vi "Power Supply (No Objects).vi"(8 "error in (no error)":errorcluster, 11 "Cluster In":T4={"Field"=0.0, "Rate"=0.0, "Status"={"Sweeping"=FALSE, "Clamped"=FALSE, "Hold"=FALSE, "At Rest"=FALSE, "Quench"=FALSE, "Persistent Mode"=FALSE, "Switch Heater"=FALSE}, "ILM Shut Down?"=FALSE, "IO Info"={"Address"={"Com Port"=1, "ISOBUS Address"=2, "GPIB Address"=24, "Communication"=enum."ISOBUS"}, "Version"=enum."IPS"}, "IO Info (Level Meter)"={"Address"={"Com Port"=1, "ISOBUS Address"=5, "GPIB Address"=24, "Communication"=enum."ISOBUS"}, "ILM Name"="", "Display Channel"=[]}, "Training?"=FALSE, "Training Field and Speed Cluster"={"Training Field"=[0.0, 4.108, 5.78, 8.001], "Training Speed"=[0.0057, 0.0022833333333333334, 0.0011333333333333334, 0.0011333333333333334]}}) -> (0 "error out":errorcluster, 3 "Cluster Out":T4={"Field"=0.0, "Rate"=0.0, "Status"={"Sweeping"=FALSE, "Clamped"=FALSE, "Hold"=FALSE, "At Rest"=FALSE, "Quench"=FALSE, "Persistent Mode"=FALSE, "Switch Heater"=FALSE}, "ILM Shut Down?"=FALSE, "IO Info"={"Address"={"Com Port"=1, "ISOBUS Address"=2, "GPIB Address"=24, "Communication"=enum."ISOBUS"}, "Version"=enum."IPS"}, "IO Info (Level Meter)"={"Address"={"Com Port"=1, "ISOBUS Address"=5, "GPIB Address"=24, "Communication"=enum."ISOBUS"}, "ILM Name"="", "Display Channel"=[]}, "Training?"=FALSE, "Training Field and Speed Cluster"={"Training Field"=[0.0, 4.108, 5.78, 8.001], "Training Speed"=[0.0057, 0.0022833333333333334, 0.0011333333333333334, 0.0011333333333333334]}})   [LabVIEW 2012]
uses:
  Magnet status.ctl
  Oxford/PSSUBS.LLB/PSIO.ctl
  Oxford/BUSGEN.LLB/OxfordAddress.ctl
  Global/GPIB Numbers.vi
  Power Supply.lvclass
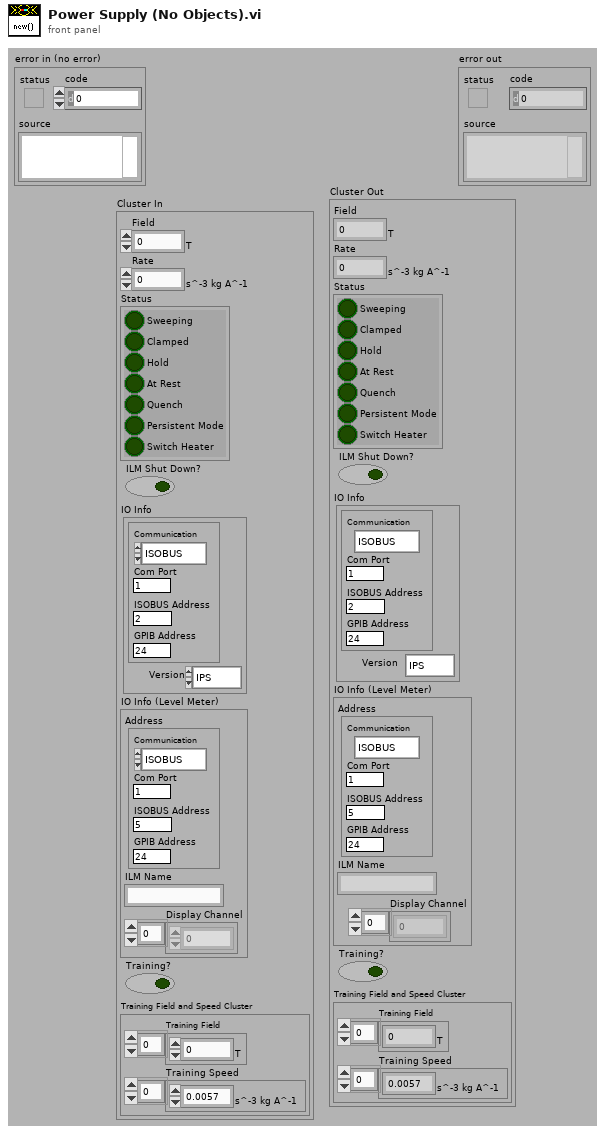
[diagram p1: front panel]
types:
  T1 = typedef "Power Supply.lvclass/Magnet status.ctl" = cluster{"Sweeping":bool, "Clamped":bool, "Hold":bool, "At Rest":bool, "Quench":bool, "Persistent Mode":bool, "Switch Heater":bool}
  T2 = typedef "PSIO.ctl" = cluster{"Address":T3, "Version":enum16{"PS", "IPS"}}
  T3 = typedef "OxfordAddress.ctl" = cluster{"Com Port":i32, "ISOBUS Address":i32, "GPIB Address":i16, "Communication":enum16{"RS232", "ISOBUS", "GPIB", "Gateway"}}
  T4 = cluster{"Field":dbl[unit], "Rate":dbl[unit], "Status":T1, "ILM Shut Down?":bool, "IO Info":T2, "IO Info (Level Meter)":cluster{"Address":T3, "ILM Name":string, "Display Channel":i32[]}, "Training?":bool, "Training Field and Speed Cluster":cluster{"Training Field":dbl[unit][], "Training Speed":dbl[unit][]}}
  T5 = cluster{"Address":T3, "ILM Name":string, "Display Channel":i32[]}
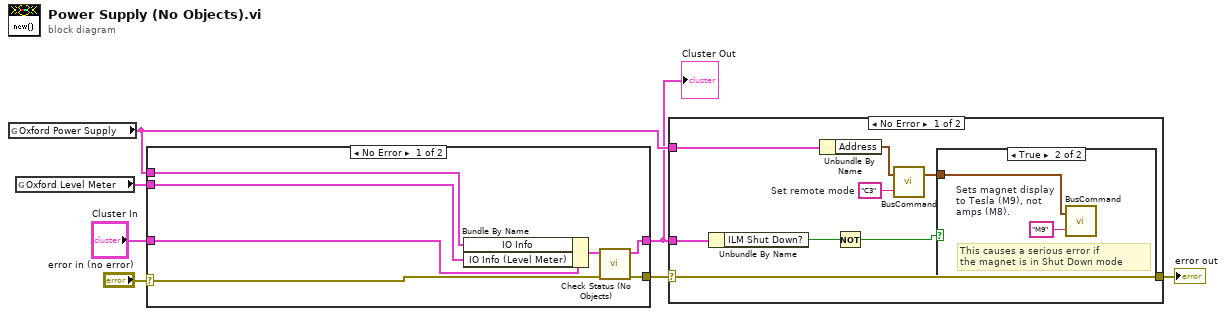
[diagram p0: block diagram]
diagram:
  n1 = global read "GPIB Numbers.vi" "Oxford Power Supply"() -> (w6:T2)
  n2 = global read "GPIB Numbers.vi" "Oxford Level Meter"() -> (w3:T5)
  n3 = case shown="No Error" "error in (no error)" {
    selector: "error in (no error)" -> [w8 w16]
    tunnel: [w13 w16] -> w5
    tunnel: [w14 w15] -> w1
    tunnel: "Cluster In" -> [w10 w15]
    tunnel: w6 -> [w12 _]
    tunnel: w3 -> [w11 _]
    frame No Error {
      n4 = Bundle By Name(cluster=w10, "IO Info"=w12, "IO Info (Level Meter)"=w11) -> (w9:T4)
      n5 = call "Check Status (No Objects).vi"("error in (no error)"=w8, "Cluster In"=w9) -> ("error out"=w13:errorcluster, "Cluster Out"=w14:T4)  [unwired: 6 in, 2 out]
    }
    frame Error {
    }
  }
  "Cluster Out" <- w1
  n6 = case shown="No Error" w5 {
    selector: w5 -> [w20 w27]
    tunnel: w6 -> [w21 _]
    tunnel: [w20 w27] -> w4
    tunnel: w1 -> [w19 _]
    frame No Error {
      w23 = "C3"  # Set remote mode
      n7 = Unbundle By Name(w19) -> ("ILM Shut Down?"=w18:bool)
      n8 = Unbundle By Name(w21) -> ("Address"=w22:T3)
      n9 = Not(x=w18) -> (.not. x?=w17:bool)
      n10 = call "BusCommand.vi"("Command"=w23, "Instrument address (in)"=w22) -> ("Instrument address (out)"=w24:T3)  [unwired: 1 out]
      n11 = case shown="True" w17 {
        tunnel: w24 -> [_ w26]
        frame False {
        }
        frame True {
          w25 = "M9"  # Sets magnet display to Tesla (M9), not  amps (M8).
          # "This causes a serious error if \nthe magnet is in Shut Down mode"
          n12 = call "BusCommand.vi"("Command"=w25, "Instrument address (in)"=w26) -> ()  [unwired: 2 out]
        }
      }
    }
    frame Error {
    }
  }
  "error out" <- w4
